vi "FPGA_main.vi"() -> ()   [LabVIEW 2010]
uses:
  <vilib>/Platform/TimedLoop/XDataNode/XDataNode.xnode
  <vilib>/Platform/TimedLoop/XDataNode/timing_clust.ctl
  <vilib>/Platform/TimedLoop/XDataNode/nitl_modes.ctl
  <vilib>/Platform/TimedLoop/XDataNode/wakeup.ctl
  <vilib>/rvi/DataTransferAndStorage/Container/XNode/niFpgaContainer.xnode
  <vilib>/rvi/DataTransferAndStorage/Container/Common/niFpgaTransferTypeControl.ctl
  <vilib>/rvi/FIFO/Fifo_Types/niFpgaFifoControlLogicControl.ctl
  <vilib>/rvi/DataTransferAndStorage/Container/Common/niFpgaContainerMethod.ctl
  <vilib>/rvi/DataTransferAndStorage/Container/Common/niFpgaContainerMetaDataKey.ctl
  <vilib>/rvi/DataTransferAndStorage/FIFO/niFpgaPeerToPeerStreamState.ctl
  <vilib>/rvi/DataTransferAndStorage/Container/Common/niFpgaContainerExecOnDevCompGetState.vi
  <vilib>/rvi/FIFO/Fifo_Resource/nirvififoEmulationSetSize.vi
  <vilib>/rvi/DataTransferAndStorage/Container/Common/niFpgaContainerGetUniqueNameForEmu.vi
  <vilib>/rvi/interface/RandomDataEmulation/nirviRandomDataFPGAFIFO.vi
  <vilib>/rvi/interface/RandomDataEmulation/niFpgaRandomDataHandleErrors.vi
  <vilib>/rvi/eio/common/nirviEmuReportErrorAndStop.vi
  <vilib>/Platform/TimedLoop/XDataNode/XDNodeRunTimeDep.lvlib
panel:
  in  "I2C clock divisor":u8=25
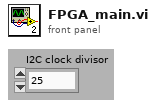
[diagram p1: front panel]
types:
  T1 = typedef "XDNodeRunTimeDep.lvlib/timing_clust.ctl" = cluster{"Expected End [f-1]":u64, "Actual End [f-1]":u64, "Finished Late? [f-1]":bool, "Expected End [i-1]":u64, "Actual End [i-1]":u64, "Finished Late? [i-1]":bool, "Expected Start [i]":u64, "Actual Start [i]":u64, "Expected Start [f]":u64, "Actual Start [f]":u64, "Source Name":string, "Structure Name":string, "Period":i64, "Deadline":i64, "Offset":i64, "Start":i64, "Priority":i32, "Timeout":i32, "Mode":T2, "Wakeup Reason":T3, "Error":errorcluster, "Source Type":string, "Secondary Source Type":string, "Global End Time":u64, "Global Start Time":u64, "Frame Duration":u64, "Iteration Duration":u64, "Assigned CPU":i32, "I/O Scan Engine Mode":u32}
  T2 = typedef "XDNodeRunTimeDep.lvlib/nitl_modes.ctl" = enum32{"No Change", "Process missed periods, maintain original phase", "Discard missed periods, maintain original phase", "Process missed periods, ignore original phase", "Discard missed periods, ignore original phase"}
  T3 = typedef "XDNodeRunTimeDep.lvlib/wakeup.ctl" = enum32{"Normal", "Aborted", "Asynchronous wakeup", "Timing source error", "Timed loop error", "Timeout"}
  T4 = typedef "niFpgaFifoControlLogicControl.ctl" = enum16{"Slice Fabric", "Target Optimal", "Built-in"}
  T5 = typedef "niFpgaContainerMethod.ctl" = enum16{"<none>", "write", "read", "clear", "getNumberOfElementsToWrite", "getNumberOfElementsToRead", "enable", "disable", "flushAndDisable", "getStreamState", "readA", "readB", "dramWrite", "dramWriteWithByteEnables", "dramRequestData", "dramRetrieveData"}
  T6 = typedef "niFpgaTransferTypeControl.ctl" = enum16{"Target-Scoped", "Host to Target - DMA", "Target to Host - DMA", "Peer to Peer Reader", "Peer to Peer Writer", "Bidirectional"}
  T7 = typedef "niFpgaPeerToPeerStreamState.ctl" = enum16{"Unlinked", "Disabled", "Enabled", "Flushing"}
  T8 = typedef "niFpgaContainerMetaDataKey.ctl" = enum16{"FPGA FIFO", "FPGA Memory", "FPGA Register"}
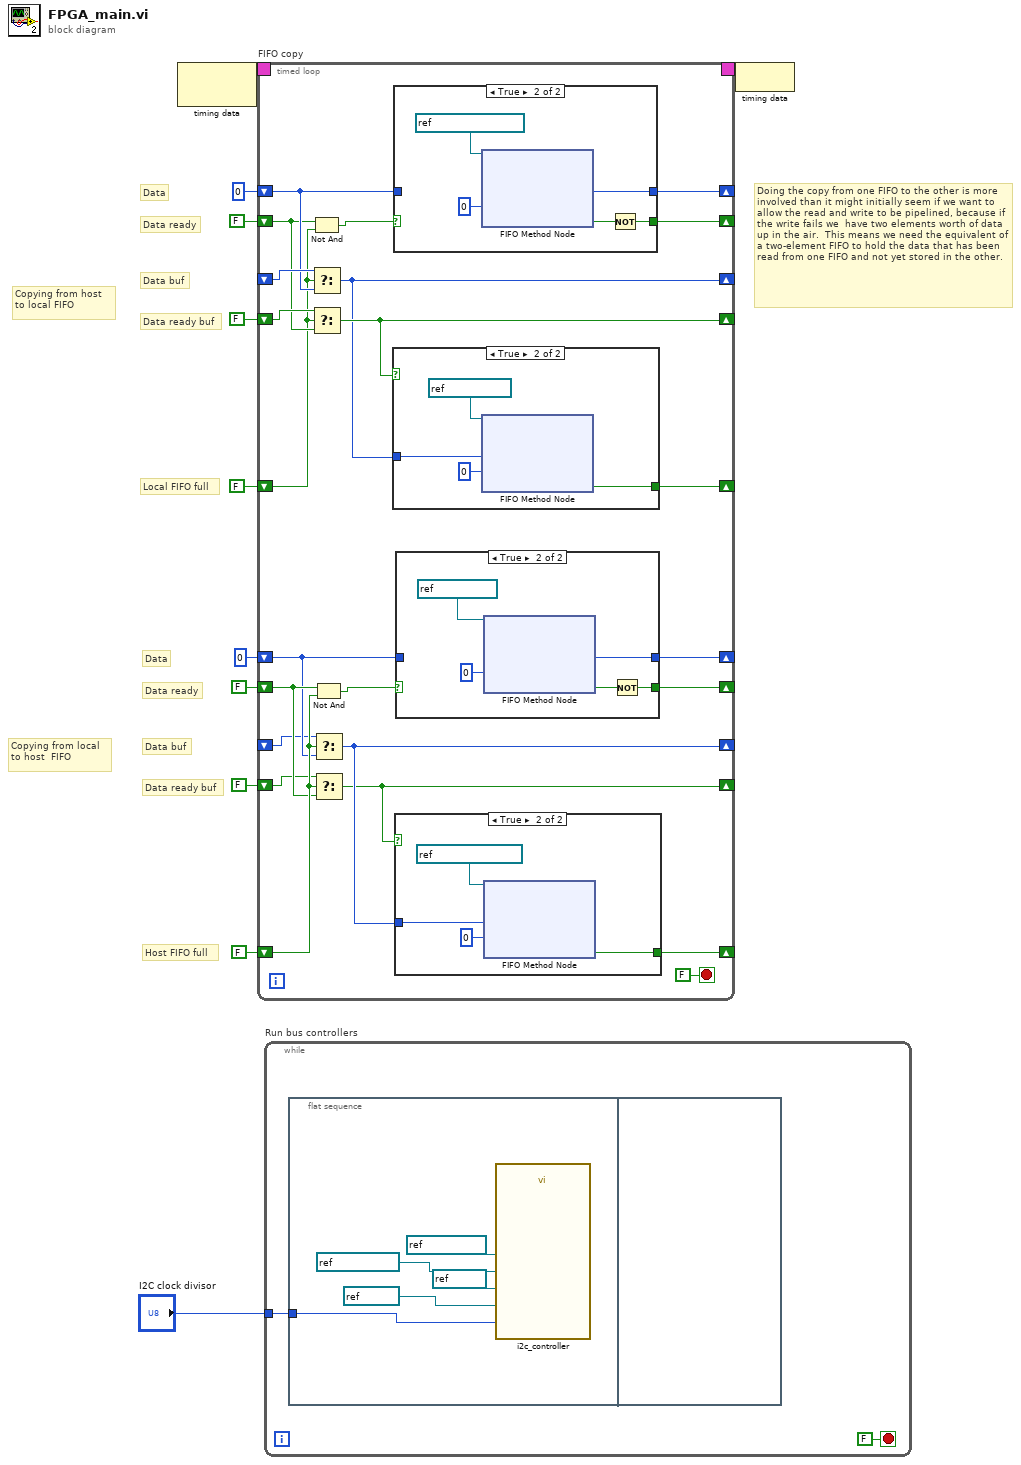
[diagram p0: block diagram]
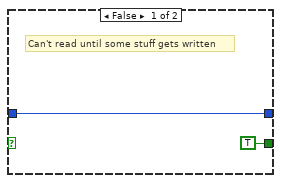
[diagram p2: hidden frame]
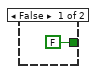
[diagram p3: hidden frame]
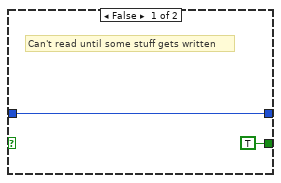
[diagram p4: hidden frame]
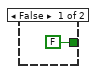
[diagram p5: hidden frame]
diagram:
  # "Copying from local to host  FIFO"
  # "Data ready buf"
  # "Data buf"
  # "Data"
  # "Data ready"
  # "Host FIFO full"
  # "Doing the copy from one FIFO to the other is more involved than it might initially seem if we want to allow the read and write to be pipelined, because if the write fails we  have two elements worth of data up in the air.  This means we need the equivalent of a two-element FIFO to hold the data that has been read from one FIFO and not yet stored in the other."
  # "Data ready buf"
  # "Data buf"
  # "Copying from host to local FIFO"
  # "Data"
  # "Data ready"
  # "Local FIFO full"
  n1 = node-c288() -> (w10:T1)  [unwired: 1 in]
  n2 = timed-loop "FIFO copy" {
    timing: w10 -> [_]
    timing-out: [_] -> w9
    shift-right: [w32] -> _
    shift-left: FALSE ("Timed Out?") -> [w26]
    shift-right: [w33] -> _
    shift-left: FALSE ("Timed Out?") -> [w27]
    shift-right: [w34] -> _
    shift-left: u8 0 ("Element") -> [w28]
    shift-right: [w23] -> _
    shift-left: _ -> [w29]
    shift-right: [w24] -> _
    shift-left: FALSE ("Timed Out?") -> [w30]
    shift-right: [w14] -> _
    shift-left: FALSE ("Timed Out?") -> [w19]
    shift-right: [w13] -> _
    shift-left: FALSE ("Timed Out?") -> [w18]
    shift-right: [w12] -> _
    shift-left: u8 0 ("Element") -> [w17]
    shift-right: [w22] -> _
    shift-left: _ -> [w16]
    shift-right: [w21] -> _
    shift-left: FALSE ("Timed Out?") -> [w15]
    stop <- FALSE stop-if-true
    n3 = Not And(1:w26, 2:w27) -> (0:w25:bool)
    n4 = Select(t=w29, s=w26, f=w28) -> (s? t:f=w23:u8)
    n5 = Select(t=w30, s=w26, f=w27) -> (s? t:f=w24:bool)
    n6 = Not And(1:w19, 2:w18) -> (0:w20:bool)
    n7 = Select(t=w16, s=w19, f=w17) -> (s? t:f=w22:u8)
    n8 = Select(t=w15, s=w19, f=w18) -> (s? t:f=w21:bool)
    n9 = case shown="True" w24 {
      tunnel: [FALSE ("Timed Out?") w1008] -> w32
      tunnel: w23 -> [_ w1006]
      frame False {
      }
      frame True {
        n10 = xnode ("FIFO Method Node")("Element"=w1006, "Timeout"=0, "FIFO In"=refnum<k21> "I2C write 0" ("FIFO")) -> ("Timed Out?"=w1008:bool)  [unwired: 1 out]
      }
    }
    n11 = case shown="True" w25 {
      tunnel: [w682 w685] -> w34
      tunnel: [TRUE w684] -> w33
      tunnel: w28 -> [w682 _]
      frame False {
        # "Can't read until some stuff gets written"
      }
      frame True {
        n12 = xnode ("FIFO Method Node")("Timeout"=0, "FIFO In"=refnum<k21> "Host write FIFO") -> ("Element"=w685:u8, "Timed Out?"=w683:bool)  [unwired: 1 out]
        n13 = Not(x=w683) -> (.not. x?=w684:bool)
      }
    }
    n14 = case shown="True" w21 {
      tunnel: [FALSE ("Timed Out?") w362] -> w14
      tunnel: w22 -> [_ w360]
      frame False {
      }
      frame True {
        n15 = xnode ("FIFO Method Node")("Element"=w360, "Timeout"=0, "FIFO In"=refnum<k21> "Host read FIFO" ("FIFO")) -> ("Timed Out?"=w362:bool)  [unwired: 1 out]
      }
    }
    n16 = case shown="True" w20 {
      tunnel: [w36 w39] -> w12
      tunnel: [TRUE w38] -> w13
      tunnel: w17 -> [w36 _]
      frame False {
        # "Can't read until some stuff gets written"
      }
      frame True {
        n17 = xnode ("FIFO Method Node")("Timeout"=0, "FIFO In"=refnum<k21> "I2C read 0") -> ("Element"=w39:u8, "Timed Out?"=w37:bool)  [unwired: 1 out]
        n18 = Not(x=w37) -> (.not. x?=w38:bool)
      }
    }
  }
  n19 = while "Run bus controllers" {
    tunnel: "I2C clock divisor" -> [w1330]
    stop <- FALSE stop-if-true
    n20 = flat-sequence {
      tunnel: w1330 -> [w1331]
      frame #0 {
        n21 = call "i2c_controller.vi"("I2C clock divisor"=w1331, "Read FIFO"=refnum<k21> "I2C read 0", "Write FIFO"=refnum<k21> "I2C write 0", "SDA out pin"=refnum<k21> "SDA0" ("SDA pin"), "SCL in pin"=refnum<k21> "SCL0" ("SCL pin")) -> ()  [unwired: 7 in]
      }
      frame #1 {
      }
    }
  }
  n22 = node-c288(w9) -> ()
